vi "OFDM-SIM-A发射机.vi"(4 "SIM比特":i32[](array[numeric]), 6 "?":T1={"过采样因子"=20.0, "脉冲成形参数"={"调制类型"=enum."PSK", "脉冲成形滤波器"=enum."Raised Cosine", "滤波器参数"=0.5, "滤波长度 (码元)"=8.0}, "载波数"=128, "总比特数"=25600, "循环次数"=1000, "信噪比门限/dB"=15, "M-QAM (16)"=4} {"脉冲成形参数"."滤波器参数" format="%.2f"}, 7 "error in (no error)":errorcluster, 8 "M-QAM (16)":i32=4, 9 "载波数":i32=128, 10 "总比特数":i32=25600) -> (0 "error out":errorcluster, 1 "输入比特流":i8[](array[numeric]) caption="output bit stream", 2 "天线2发射信号":cdb[](array[numeric]), 3 "天线1发射信号":cdb[](array[numeric]), 5 "理论4QAM星座图":cdb[](graph))   [LabVIEW 2018]
uses:
  <vilib>/Analysis/2dsp.llb/Inverse Complex FFT.vi
  <vilib>/Analysis/NI_AALPro.lvlib
panel:
  out "相位 2":dbl[](graph)
  out "频域波形(FFT) 2":dbl[](graph)
  out "相位":dbl[](graph)
  out "频域波形(FFT)":dbl[](graph)
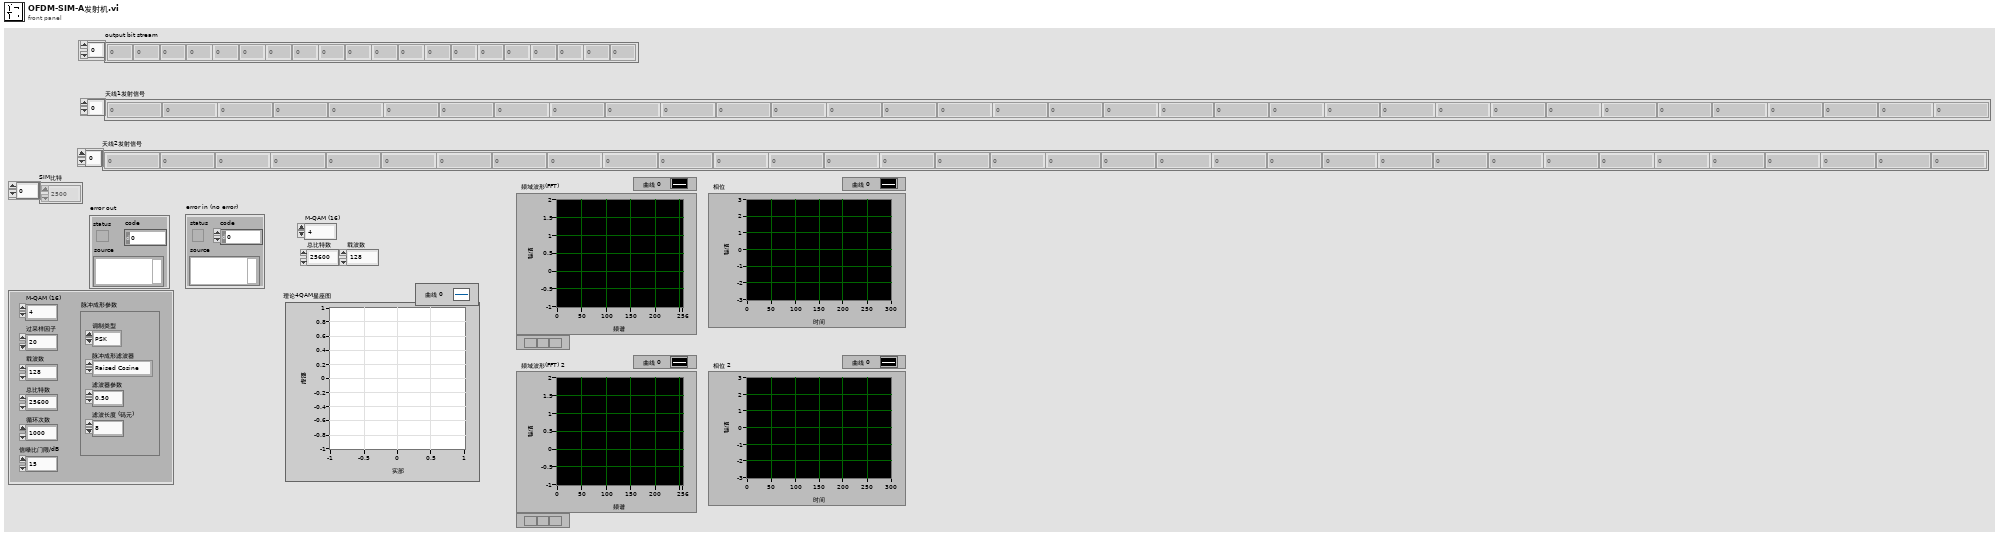
[diagram p1: front panel]
types:
  T1 = cluster{"过采样因子":dbl, "脉冲成形参数":cluster{"调制类型":enum16{"FSK", "PSK", "QAM", "MSK", "PAM", "ASK", "CPM"}, "脉冲成形滤波器":enum16{"none", "Raised Cosine", "Root Raised Cos", "Gaussian"}, "滤波器参数":dbl, "滤波长度 (码元)":dbl}, "载波数":i32, "总比特数":i32, "循环次数":i32, "信噪比门限/dB":i32, "M-QAM (16)":i32}
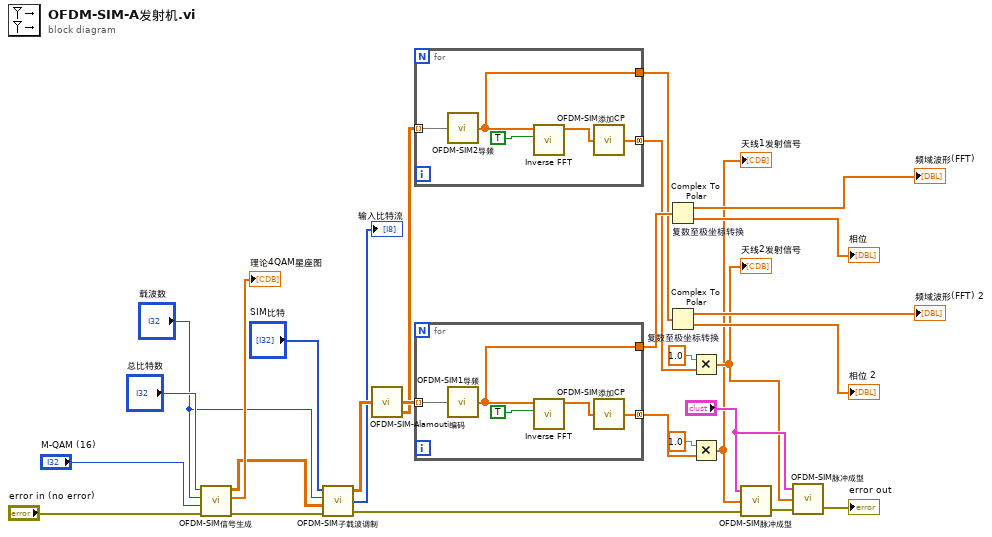
[diagram p0: block diagram]
diagram:
  n1 = call "OFDM-SIM信号生成.vi"("总比特数"="总比特数", "载波数"="载波数", "M-QAM"="M-QAM (16)", "error in (no error)"="error in (no error)") -> ("并行信号"=w6:cdb[][], "理论4QAM星座图"=→"理论4QAM星座图":cdb[], "error out"=w8:errorcluster)  [unwired: 2 out]
  n2 = call "OFDM-SIM子载波调制.vi"("error in"=w8, "并行信号"=w6, "载波数"="载波数", "SIM比特"="SIM比特") -> ("error out"=w4:errorcluster, "实际输入序列"=→"输入比特流":i32[], "SIM输出"=w7:cdb[][])
  n3 = call "OFDM-SIM-Alamouti编码.vi"("调制符号流"=w7) -> ("天线1信号"=w13:cdb[][], "天线2信号"=w12:cdb[][])  [unwired: 1 out]
  n4 = for {
    tunnel: w12 -> [w32] mode=indexing
    tunnel: [w29] -> w19 mode=concatenating
    tunnel: [w31] -> w23
    n5 = call "OFDM-SIM2导频.vi"("输入的OFDM符号"=w32) -> ("OFDM-IM output"=w31:cdb[])
    n6 = call-poly <vilib>:"Inverse FFT.vi"("shift?"=TRUE, "FFT {X}"=w31) -> ("X"=w30:cdb[])  [unwired: 8 in, 1 out]
    n7 = call "OFDM-SIM添加CP.vi"("输入符号"=w30) -> ("加CP后"=w29:cdb[])
  }
  n8 = for {
    tunnel: w13 -> [w37] mode=indexing
    tunnel: [w35] -> w24 mode=concatenating
    tunnel: [w36] -> w28
    n9 = call "OFDM-SIM1导频.vi"("输入的OFDM符号"=w37) -> ("OFDM-IM output"=w36:cdb[])
    n10 = call-poly <vilib>:"Inverse FFT.vi"("shift?"=TRUE, "FFT {X}"=w36) -> ("X"=w34:cdb[])  [unwired: 8 in, 1 out]
    n11 = call "OFDM-SIM添加CP.vi"("输入符号"=w34) -> ("加CP后"=w35:cdb[])
  }
  n12 = Complex To Polar "复数至极坐标转换"(r * e^(i*theta)=w28) -> (r=→"频域波形(FFT)":dbl[], theta=→"相位":dbl[])
  n13 = Complex To Polar "复数至极坐标转换"(r * e^(i*theta)=w23) -> (r=→"频域波形(FFT) 2":dbl[], theta=→"相位 2":dbl[])
  n14 = Multiply(x=1.0, y=w19) -> (x*y=w2:cdb[])
  "天线2发射信号" <- w2
  n15 = Multiply(x=1.0, y=w24) -> (x*y=w1:cdb[])
  "天线1发射信号" <- w1
  n16 = call "OFDM-SIM脉冲成型.vi"("error in (no error)"=w4, "输入"=w1, 4:"?") -> ("error out"=w3:errorcluster)  [unwired: 1 out]
  n17 = call "OFDM-SIM脉冲成型.vi"("error in (no error)"=w3, "输入"=w2, 4:"?") -> ("error out"=→"error out":errorcluster)  [unwired: 1 out]
